vi "P0.5_XY_Digital.vi"(11 "In":waveform(dbl)) -> (2 "P0.5_Digital_XY":digitalwaveform(waveform)={"t0"=timestamp(0 s since 1904-01-01), "dt"=0.0, "Y"={"transitions"=[], "data"=[]}, "error"={"status"=FALSE, "code"=37421928, "source"=""}}, 3 "Out":waveform(dbl))   [LabVIEW 2018]
uses:
  <vilib>/Waveform/DWDTOps.llb/DWDT Analog to Digital.vi
  <vilib>/measure/NI_MABase.lvlib
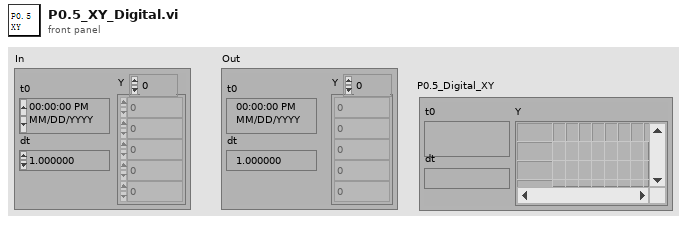
[diagram p1: front panel]
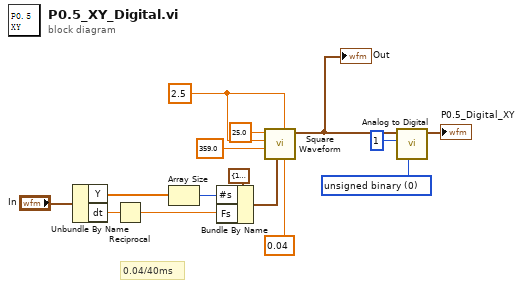
[diagram p0: block diagram]
diagram:
  w2 = u16 0 items=["unsigned binary", "offset binary", "2's complement"] ("data format (offset binary)")
  w6 = 2.5 ("offset")
  # "0.04/40ms"
  n1 = Unbundle By Name("In") -> ("Y"=w9:dbl[], "dt"=w13:dbl)
  n2 = Reciprocal(x=w13) -> (1/x=w14:dbl)
  n3 = Array Size(array=w9) -> (size(s)=w12:i32)
  n4 = Bundle By Name(cluster=cluster{"Fs":dbl, "#s":dbl} {"Fs"=1000.0, "#s"=1000.0} ("sampling info"), "#s"=w12, "Fs"=w14) -> (w11:cluster{"Fs":dbl, "#s":dbl})
  n5 = call <vilib>:"Square Waveform.vi"("duty cycle (%)"=0.04, "offset"=w6, "sampling info"=w11, "phase"=359.0, "amplitude"=w6, "frequency"=25.0) -> ("signal out"=w3:waveform(dbl))  [unwired: 4 in, 1 out]
  "Out" <- w3
  n6 = call-poly <vilib>:"Analog to Digital.vi"("data format (offset binary)"=w2, "resolution (16 bit)"=1, "analog waveform"=w3) -> ("digital waveform"=→"P0.5_Digital_XY":digitalwaveform)  [unwired: 5 in, 3 out]
